vi "testLuaL_Buffer.vi"() -> ()   [LabVIEW 2011]
panel:
  out "Modified_LuaL_Buffer":T1 {"char *b" format="%x"; "size_t size" format="%x"; "lua_State *L" format="%x"}
  out "luaL_Buffer *B 2":T1 {"char *b" format="%x"; "size_t size" format="%x"; "lua_State *L" format="%x"}
  out "luaL_Buffer *B":T1 {"char *b" format="%x"; "size_t size" format="%x"; "lua_State *L" format="%x"}
  in  "size_t l":i32
  in  "const char *s":string
  in  "lua_State *L":u64
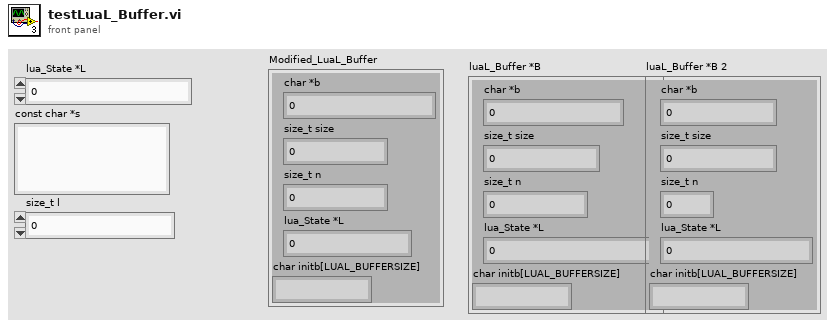
[diagram p1: front panel]
types:
  T1 = cluster{"char *b":u32, "size_t size":u32, "size_t n":u32, "lua_State *L":u64, "char initb[LUAL_BUFFERSIZE]":string}
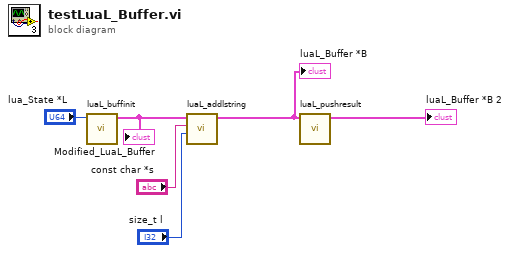
[diagram p0: block diagram]
diagram:
  n1 = call "luaL_buffinit.vi"("lua_State *L"="lua_State *L") -> ("Modified_LuaL_Buffer"=w5:T1)  [unwired: 9 in, 1 out]
  "Modified_LuaL_Buffer" <- w5
  n2 = call "luaL_addlstring.vi"("size_t l"="size_t l", "const char *s"="const char *s", "luaL_Buffer *B input"=w5) -> ("luaL_Buffer *B"=w2:T1)  [unwired: 7 in, 1 out]
  "luaL_Buffer *B" <- w2
  n3 = call "luaL_pushresult.vi"("luaL_Buffer *B input"=w2) -> ("luaL_Buffer *B"=→"luaL_Buffer *B 2":T1)  [unwired: 9 in, 1 out]
